vi "Test AO.vi"() -> ()   [LabVIEW 2013]
uses:
  <vilib>/FPGAPlugInAG/PXIe-7962R/niLvFpga_Open_PXIe-7962R.vi
  <vilib>/rvi/interface/common/dynamic/niFpgaDynamicAddResources.vi
  <vilib>/FPGAPlugInAG/Dynamic/niLvFpga_Abort_Dynamic.vi
  <vilib>/FPGAPlugInAG/Dynamic/niLvFpga_Reset_Dynamic.vi
  <vilib>/rvi/interface/common/niFpgaWaitOnOcc.vi
  <vilib>/Utility/error.llb/Error Cluster From Error Code.vi
  <vilib>/FPGAPlugInAG/Dynamic/niLvFpga_Run_Dynamic.vi
  <vilib>/rvi/errors/niLvFpgaAdjustHostInterfaceError.vi
  <vilib>/FPGAPlugInAG/Dynamic/niLvFpga_Close_Dynamic.vi
  <vilib>/rvi/interface/nirviOpenFPGA/nirviOpenFPGA.xnode
  FPGA Bitfiles/LIDAR Module 5782 V3.3.lvbitx
  <vilib>/rvi/interface/nirviMethod/nirviMethod.xnode
  <vilib>/rvi/interface/nirviReadWriteControl/nirviReadWriteControl.xnode
  <vilib>/rvi/interface/nirviCloseFPGA/nirviCloseFPGA.xnode
  <vilib>/rvi/errors/niLvFpgaMergeErrorWithErrorCode.vi
  <vilib>/rvi/interface/Simulation/niFpgaSimulationCallBeginRW.vi
  NiFpgaLv.dll
  <vilib>/FPGAPlugInAG/Dynamic/niLvFpga_StopFifo_Dynamic.vi
  <vilib>/FPGAPlugInAG/Dynamic/niLvFpga_ConfigureFifo_Dynamic.vi
  <vilib>/FPGAPlugInAG/Dynamic/niLvFpga_AcquireReadRegionFifo_Dynamic.vi
panel:
  in  "StreamToDMA":bool
  out "Elements Remaining":u32
  out "Numeric":i32=89152
  in  "Write To File":bool
  out "Numeric 2":dbl=375.0
  in  "Elements":u32=100000
  out "error out 3":errorcluster
  out "error out 2":errorcluster
  in  "file path (use dialog)":path=path "C:/Users/LIDAR/Desktop/Scans/InterScan4.dat"
  out "Actual Depth":u32=400384
  out "Timeouts":u16
  in  "SamplingEnable":bool
  in  "SingleFrame":bool
  in  "NoOfLeds":u16=319
  in  "PulseWaitClck":u8=40
  in  "PulseUpClck":u8=5
  in  "LaserPower 0":bool=TRUE
  in  "LaserPower 1":bool=TRUE
  in  "LedScanDebEn":bool
  in  "ActiveLedIndexDeb":u16
  out "error out":errorcluster
  in  "stop":bool=TRUE
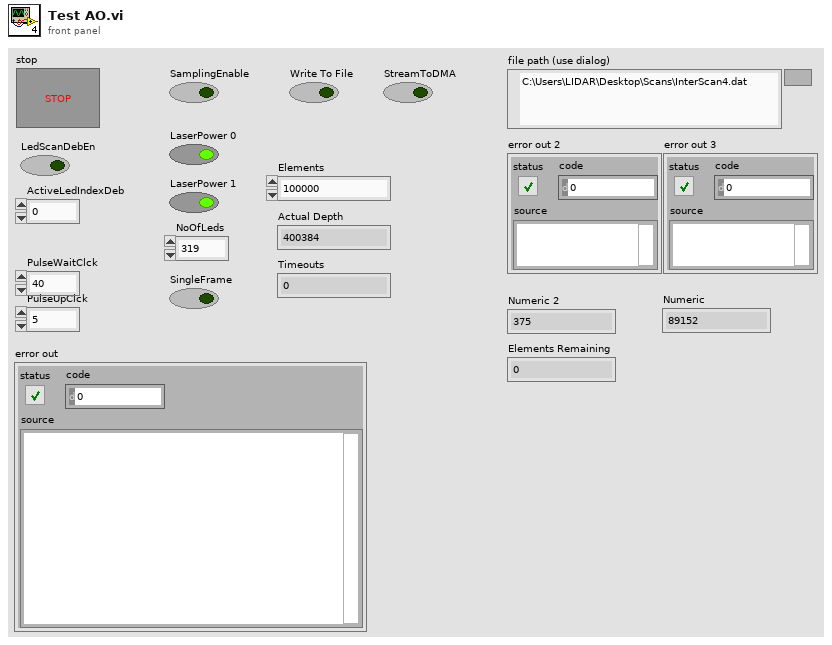
[diagram p1: front panel]
types:
  T1 = enum16{"open", "replace", "create", "open or create", "replace or create", "replace or create with confirmation"}
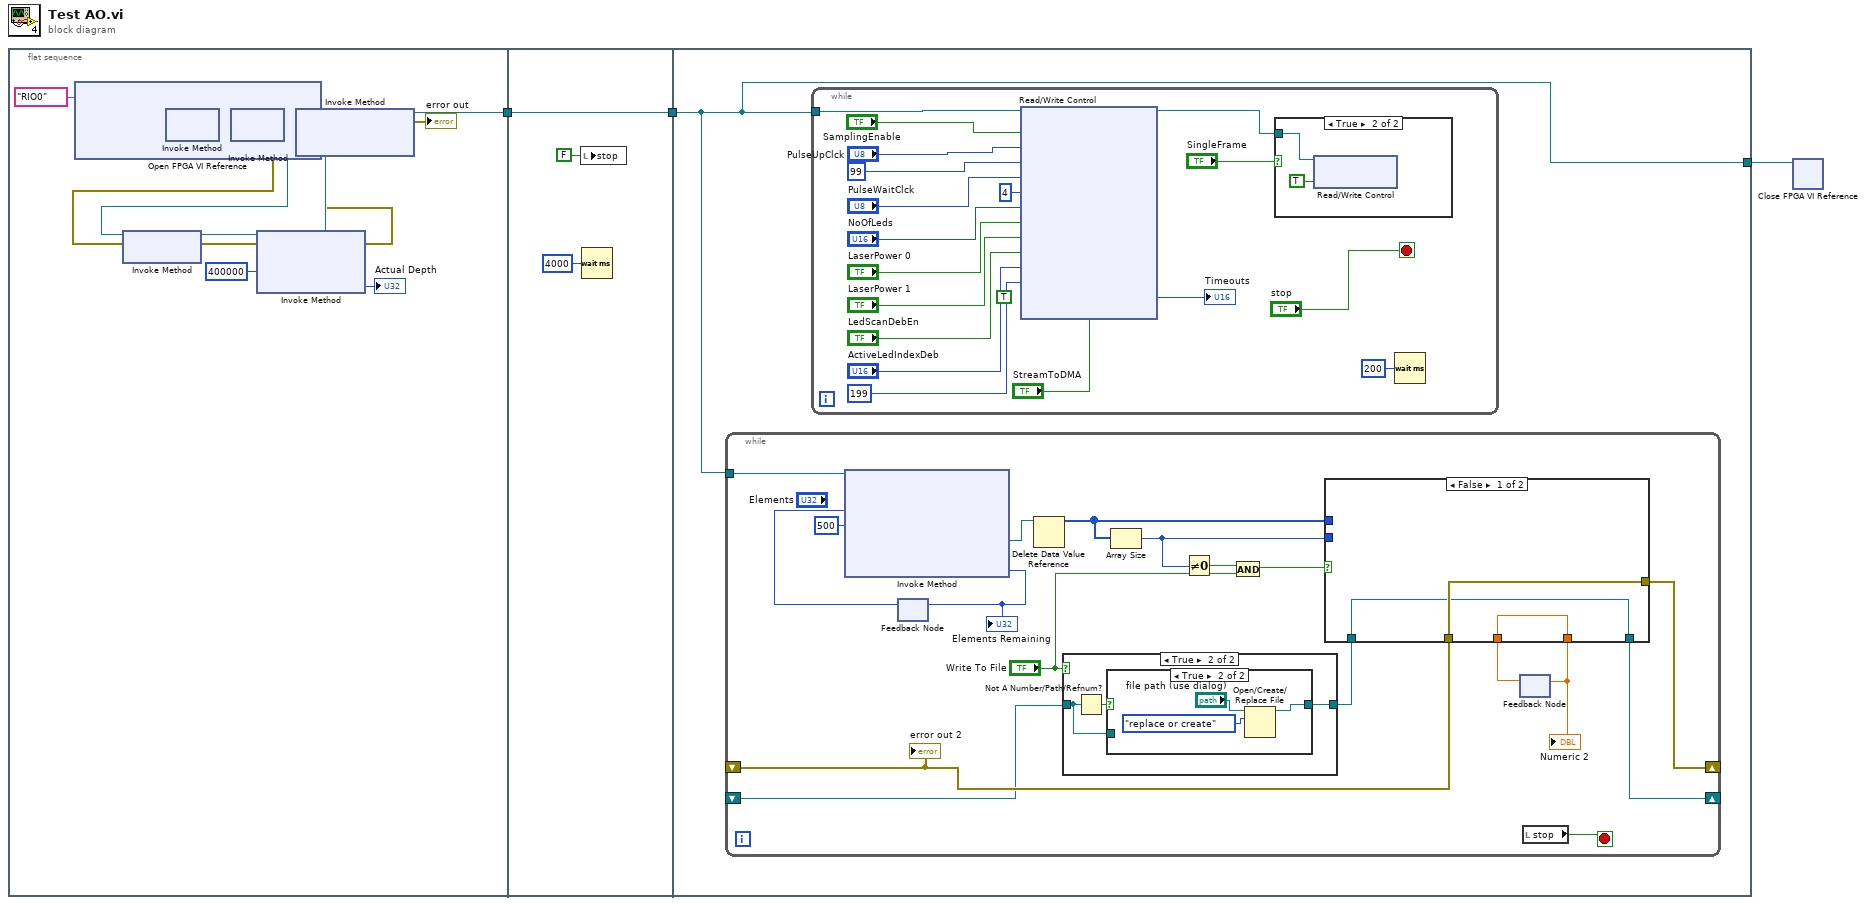
[diagram p0: block diagram]
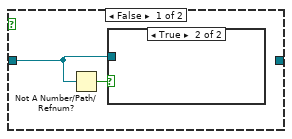
[diagram p2: hidden frame]
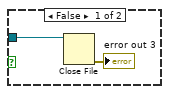
[diagram p3: hidden frame]
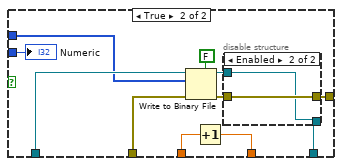
[diagram p5: hidden frame]
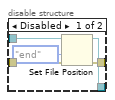
[diagram p6: hidden frame]
diagram:
  n1 = flat-sequence {
    tunnel: [w13] -> w2
    tunnel: [w19] -> w3
    tunnel: w2 -> [w19]
    tunnel: w3 -> [w22]
    tunnel: [w22] -> w1
    frame #0 {
      n2 = xnode "Open FPGA VI Reference"("resource name"=tag "RIO0") -> ("FPGA VI Reference Out"=w14:refnum<k20>, "error out"=w15:errorcluster)  [unwired: 1 in]
      n3 = xnode "Invoke Method"("FPGA VI Reference In"=w14, "error in"=w15) -> ("FPGA VI Reference Out"=w17:refnum<k20>, "error out"=w18:errorcluster)
      n4 = xnode "Invoke Method"("FPGA VI Reference In"=w17, "error in"=w18) -> ("FPGA VI Reference Out"=w12:refnum<k20>, "error out"=w9:errorcluster)
      n5 = xnode "Invoke Method"("FPGA VI Reference In"=w12, "error in"=w9) -> ("FPGA VI Reference Out"=w10:refnum<k20>, "error out"=w11:errorcluster)
      n6 = xnode "Invoke Method"("FPGA VI Reference In"=w10, "error in"=w11, "Requested Depth"=u32 400000) -> ("FPGA VI Reference Out"=w7:refnum<k20>, "error out"=w5:errorcluster, "Actual Depth"=→"Actual Depth":u32)
      n7 = xnode "Invoke Method"("FPGA VI Reference In"=w7, "error in"=w5) -> ("FPGA VI Reference Out"=w13:refnum<k20>, "error out"=→"error out":errorcluster)  [unwired: 1 in]
    }
    frame #1 {
      n8 = local write "stop"(FALSE ("stop")) -> ()
      n9 = Wait (ms)(milliseconds to wait=u32 4000) -> ()  [unwired: 1 out]
    }
    frame #2 {
      n10 = while {
        tunnel: w22 -> [w40]
        shift-right: [w38] -> _
        shift-left: _ -> [w31]
        shift-right: [w37] -> _
        shift-left: _ -> [w36]
        stop <- w39 stop-if-true
        n11 = feedback #1() -> (w23:u32)  [unwired: 1 in]
        n12 = xnode "Invoke Method"("FPGA VI Reference In"=w40, "Number of Elements"=w23, "Timeout (ms)"=500) -> ("Read Region Reference"=w33:refnum<data-value>, "Elements Remaining"=w24:u32)  [unwired: 1 in, 3 out]
        "Elements Remaining" <- w24
        n13 = feedback-in #1(w24) -> ()
        n14 = Delete Data Value Reference(data value reference=w33) -> (data value=w27:u32[])  [unwired: 1 in, 1 out]
        n15 = case shown="True" "Write To File" {
          tunnel: w31 -> [w41 w45]
          tunnel: [_ w47] -> w30
          frame False {
            n16 = Not A Number/Path/Refnum?(number/path/refnum=w41) -> (NaN/Path/Refnum?=w42:bool)
            n17 = case shown="True" w42 {
              tunnel: w41 -> [w44 _]
              frame False {
                n18 = Close File(refnum=w44) -> (error out=→"error out 3":errorcluster)  [unwired: 1 in, 1 out]
              }
              frame True {
              }
            }
          }
          frame True {
            n19 = Not A Number/Path/Refnum?(number/path/refnum=w45) -> (NaN/Path/Refnum?=w46:bool)
            n20 = case shown="True" w46 {
              tunnel: [w48 w49] -> w47
              tunnel: w45 -> [w48 _]
              frame False {
              }
              frame True {
                n21 = Open/Create/Replace File(file path (use dialog)="file path (use dialog)", operation (0:open)=T1."replace or create") -> (refnum out=w49:refnum<file>)  [unwired: 4 in, 2 out]
              }
            }
          }
        }
        n22 = Array Size(array=w27) -> (size(s)=w26:i32)
        n23 = Not Equal To 0?(x=w26) -> (x != 0?=w25:bool)
        n24 = And(x=w25, y="Write To File") -> (x .and. y?=w32:bool)
        n25 = feedback #2() -> (w34:dbl)  [unwired: 1 in]
        n26 = case shown="False" w32 {
          tunnel: [w52 w62] -> w38
          tunnel: w36 -> [w54 w57]
          tunnel: [w54 w61] -> w37
          tunnel: [w53 w59] -> w35
          tunnel: w34 -> [w53 w60]
          tunnel: w27 -> [_ w56]
          tunnel: w30 -> [w52 w58]
          tunnel: w26 -> [_ w55]
          frame False {
          }
          frame True {
            n27 = Write to Binary File(file (use dialog)=w58, data=w56, error in=w57, 5:FALSE ("prepend array or string size? (T)")) -> (refnum out=w64:refnum<file>, error out=w65:errorcluster)  [unwired: 2 in, 1 out]
            n28 = Increment(x=w60) -> (x+1=w59:dbl)
            n29 = disable-structure shown="Enabled" {
              disable-tunnel: w65 -> [w70 w72]
              disable-tunnel: w64 -> [w68 w71]
              disable-tunnel: [w67 w71] -> w62
              disable-tunnel: [w66 w72] -> w61
              frame Disabled {
                n30 = Set File Position(refnum=w68, from (0:start)=enum16{"start", "end", "current"}."end", error in=w70) -> (refnum out=w67:refnum<file>, error out=w66:errorcluster)  [unwired: 1 in]
              }
              frame Enabled {
              }
            }
            "Numeric" <- w55
          }
        }
        "Numeric 2" <- w35
        n31 = feedback-in #2(w35) -> ()
        n32 = local read "stop"() -> (w39:bool)
        "error out 2" <- w36
      }
      n33 = while {
        tunnel: w22 -> [w90]
        stop <- "stop" stop-if-true
        (unwired) TRUE ("EnAI")
        n34 = xnode "Read/Write Control"("FPGA VI Reference In"=w90, "SamplingEnable"="SamplingEnable", "PulseEndClck"="PulseUpClck", "SampPerPulse"=u8 99, "PulseWaitClck"="PulseWaitClck", "WaitForPulseEndDelay"=u8 4, "NoOfLeds"="NoOfLeds", "PFI2"="LaserPower 0", "PFI3"="LaserPower 1", "LedScanDebEn"="LedScanDebEn", "ActiveLedIndexDeb"="ActiveLedIndexDeb", "PulsePerLed"=i16 199, "StreamToDMA"="StreamToDMA") -> ("FPGA VI Reference Out"=w81:refnum<k20>, "Timeouts"=→"Timeouts":u16)  [unwired: 1 in, 1 out]
        n35 = case shown="True" "SingleFrame" {
          tunnel: w81 -> [_ w92]
          frame False {
          }
          frame True {
            n36 = xnode "Read/Write Control"("FPGA VI Reference In"=w92, "SingleFrame"=TRUE) -> ()  [unwired: 1 in, 2 out]
          }
        }
        n37 = Wait (ms)(milliseconds to wait=u32 200) -> ()  [unwired: 1 out]
      }
    }
  }
  n38 = xnode "Close FPGA VI Reference"("FPGA VI Reference In"=w1) -> ()  [unwired: 1 in, 1 out]
